vi "SetPIDGains.vi"(10 "pidGains":dbl[](array[numeric]), 11 "Constants LL in":T1) -> (3 "Constants LL out":T1)   [LabVIEW 2024]
uses:
  typeDef/constants_LL.ctl
  GlobalVariables.vi
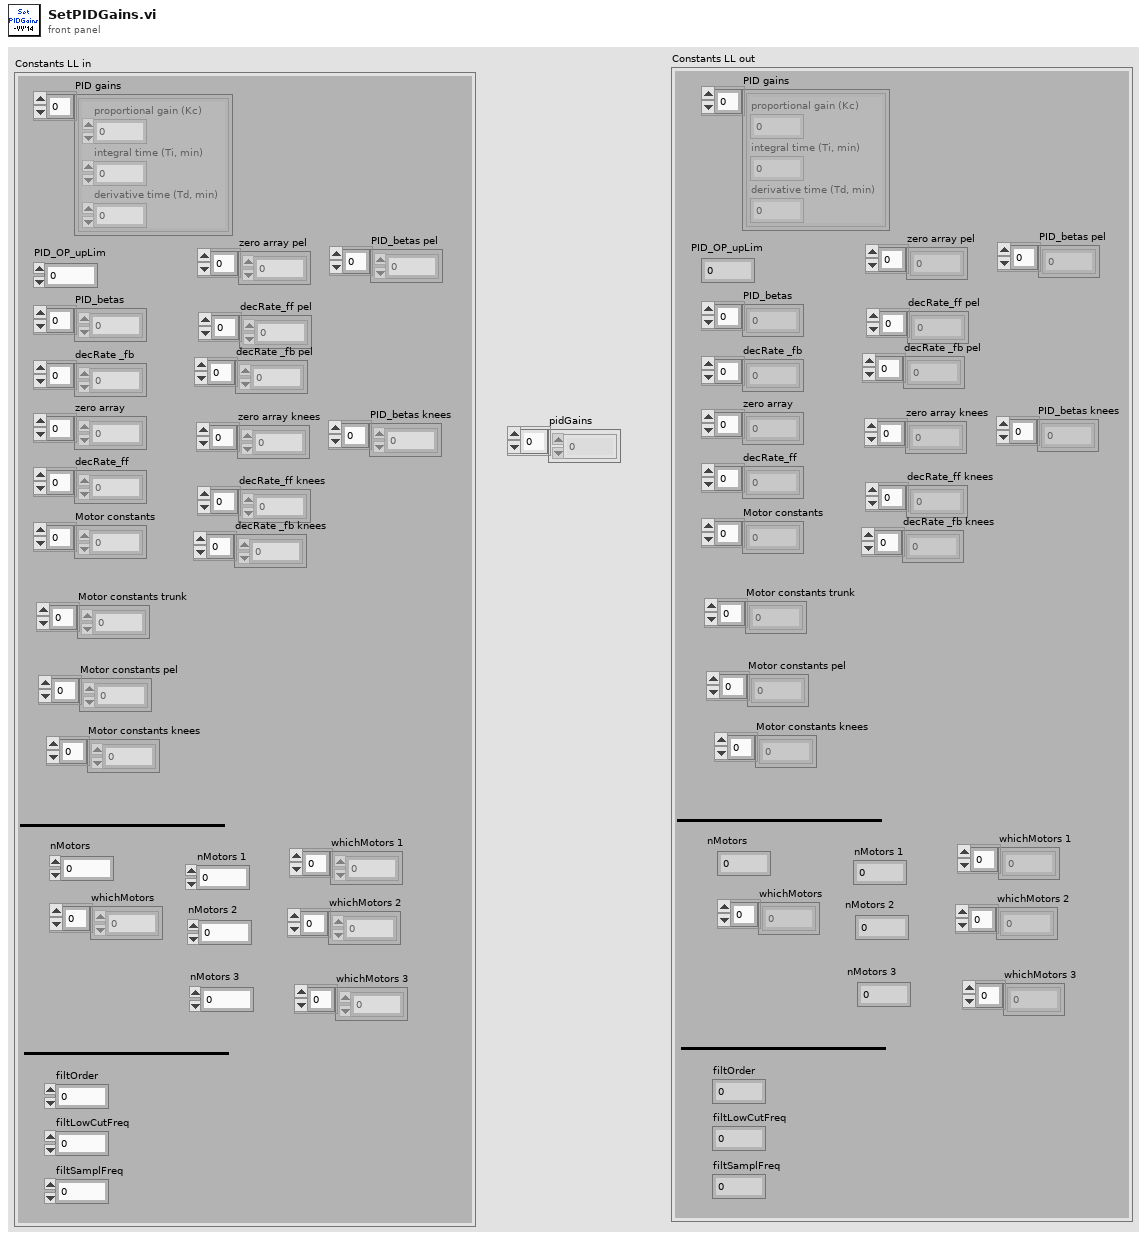
[diagram p1: front panel]
types:
  T1 = typedef "constants_LL.ctl" = cluster{"zero array":dbl[], "decRate_ff":dbl[], "Motor constants":dbl[], "PID gains":cluster{"proportional gain (Kc)":dbl, "integral time (Ti, min)":dbl, "derivative time (Td, min)":dbl}[], "decRate _fb":dbl[], "PID_OP_upLim":dbl, "nMotors":i32, "PID_betas":dbl[], "filtOrder":i32, "filtLowCutFreq":dbl, "filtSamplFreq":dbl, "whichMotors":i32[], "nMotors 1":i32, "nMotors 2":i32, "Motor constants pel":dbl[], "Motor constants trunk":dbl[], "whichMotors 1":i32[], "whichMotors 2":i32[], "zero array pel":dbl[], "decRate_ff pel":dbl[], "decRate _fb pel":dbl[], "PID_betas pel":dbl[], "whichMotors 3":i32[], "nMotors 3":i32, "Motor constants knees":dbl[], "zero array knees":dbl[], "decRate_ff knees":dbl[], "decRate _fb knees":dbl[], "PID_betas knees":dbl[]}
  T2 = cluster{"Numeric":dbl, "Numeric":dbl, "Numeric":dbl}
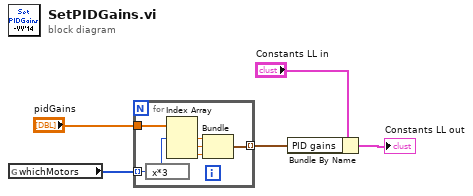
[diagram p0: block diagram]
diagram:
  n1 = global read "GlobalVariables.vi" "whichMotors"() -> (w4:i32[])
  n2 = for {
    tunnel: w4 -> [w7] mode=indexing
    tunnel: "pidGains" -> [w12]
    tunnel: [w6] -> w3 mode=indexing
    n3 = expression code="x*3"(w7) -> (w8:i32)
    n4 = Index Array(array=w12, index #1=w8) -> (element #1=w11:dbl, element #2=w10:dbl, element #3=w9:dbl)  [unwired: 2 in]
    n5 = Bundle("Numeric"=w11, "Numeric"=w10, "Numeric"=w9) -> (w6:T2)  [unwired: 1 in]
  }
  n6 = Bundle By Name(cluster="Constants LL in", "PID gains"=w3) -> (→"Constants LL out":T1)
